vi "algoritmo.vi"(3 "AH":dbl, 4 "DEC":dbl, 5 "Latitude Local":dbl) -> (0 "Altura":dbl, 1 "Módulo da Altura":dbl, 2 "Azimute":dbl)   [LabVIEW 2012]
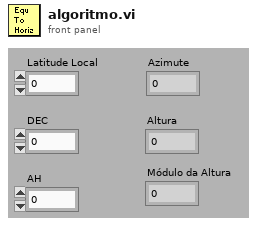
[diagram p1: front panel]
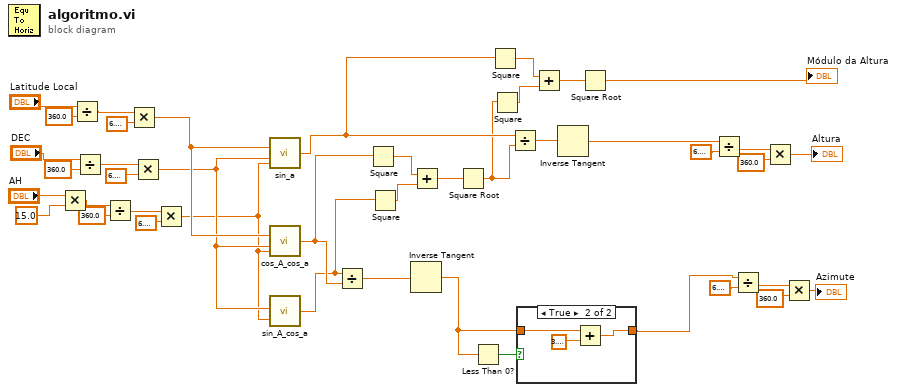
[diagram p0: block diagram]
diagram:
  n1 = Multiply(x="AH", y=15.0) -> (x*y=w15:dbl)
  n2 = Divide(x="Latitude Local", y=360.0) -> (x/y=w20:dbl)
  n3 = Divide(x="DEC", y=360.0) -> (x/y=w17:dbl)
  n4 = Divide(x=w15, y=360.0) -> (x/y=w14:dbl)
  n5 = Multiply(x=w20, y=6.283185307179586) -> (x*y=w19:dbl)
  n6 = Multiply(x=w17, y=6.283185307179586) -> (x*y=w16:dbl)
  n7 = Multiply(x=w14, y=6.283185307179586) -> (x*y=w13:dbl)
  n8 = call "sin_a.vi"("AH"=w13, "DEC"=w16, "Latitude Local"=w19) -> ("sina"=w31:dbl)
  n9 = call "cos_A_cos_a.vi"("AH"=w13, "DEC"=w16, "Latitude Local"=w19) -> ("CosAcosa"=w41:dbl)
  n10 = call "sin_A_cos_a.vi"("AH"=w13, "DEC"=w16) -> ("sinAcosa"=w40:dbl)
  n11 = Divide(x=w40, y=w41) -> (x/y=w42:dbl)
  n12 = Square(x=w41) -> (x^2=w38:dbl)
  n13 = Square(x=w40) -> (x^2=w37:dbl)
  n14 = Inverse Tangent(1:w42) -> (0:w2:dbl)
  n15 = Add(x=w38, y=w37) -> (x+y=w39:dbl)
  n16 = Square Root(x=w39) -> (sqrt(x)=w30:dbl)
  n17 = Less Than 0?(x=w2) -> (x < 0?=w3:bool)
  n18 = Square(x=w31) -> (x^2=w33:dbl)
  n19 = Square(x=w30) -> (x^2=w34:dbl)
  n20 = Divide(x=w31, y=w30) -> (x/y=w36:dbl)
  n21 = case shown="True" w3 {
    tunnel: w2 -> [w43 w45]
    tunnel: [w43 w46] -> w1
    frame False {
    }
    frame True {
      n22 = Add(x=w45, y=3.141592653589793) -> (x+y=w46:dbl)
    }
  }
  n23 = Add(x=w33, y=w34) -> (x+y=w32:dbl)
  n24 = Inverse Tangent(1:w36) -> (0:w35:dbl)
  n25 = Square Root(x=w32) -> (sqrt(x)=→"Módulo da Altura":dbl)
  n26 = Divide(x=w35, y=6.283185307179586) -> (x/y=w10:dbl)
  n27 = Divide(x=w1, y=6.283185307179586) -> (x/y=w8:dbl)
  n28 = Multiply(x=w10, y=360.0) -> (x*y=→"Altura":dbl)
  n29 = Multiply(x=w8, y=360.0) -> (x*y=→"Azimute":dbl)
